vi "Read Value.vi"(8 "error in (no error)":errorcluster, 11 "int32 in":refnum<class "int64.lvclass">) -> (0 "error out":errorcluster, 2 "Value":i64, 3 "int32 out":refnum<class "int64.lvclass">)   [LabVIEW 2020, in "Protobuf RAW.lvlib" / "int64.lvclass"]
uses:
  int64.lvclass
  int64.lvclass/int64.ctl
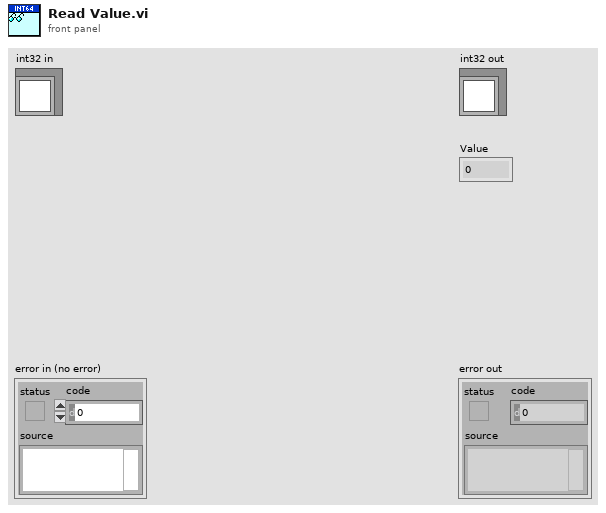
[diagram p1: front panel]
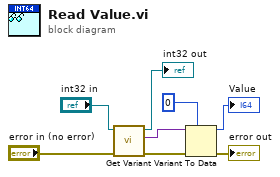
[diagram p0: block diagram]
diagram:
  n1 = call-dynamic "Get Variant.vi"("error in (no error)"="error in (no error)", "Proto Type Common in"="int32 in") -> ("error out"=w2:errorcluster, "Value"=w3:variant, "Proto Type Common out"=→"int32 out":refnum<class "int64.lvclass">)  [unwired: 7 in]
  n2 = Variant To Data(error in=w2, type=i64 0 ("Value"), Variant=w3) -> (data=→"Value":i64, error out=→"error out":errorcluster)
